vi "ci-script.vi"() -> ()   [LabVIEW 2018]
panel:
  out "error message":string
  out "Exit code":i32
  in  "arguments":string[](array[string])
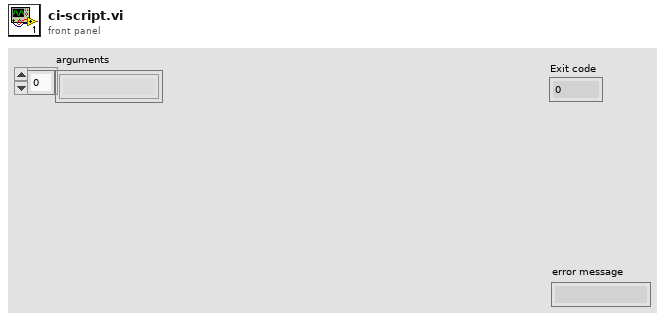
[diagram p1: front panel]
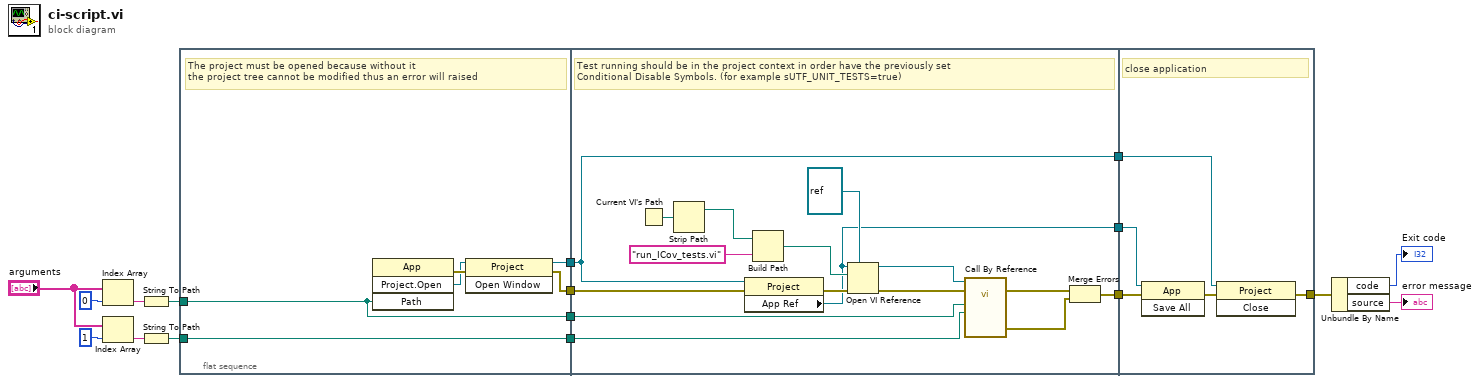
[diagram p0: block diagram]
diagram:
  n1 = Index Array(array="arguments", index=0) -> (element=w9:string)
  n2 = Index Array(array="arguments", index=1) -> (element=w7:string)
  n3 = String To Path(string=w9) -> (path=w5:path)
  n4 = String To Path(string=w7) -> (path=w4:path)
  n5 = flat-sequence {
    tunnel: w4 -> [w23]
    tunnel: w5 -> [w18]
    tunnel: [w23] -> w17
    tunnel: [w20] -> w16
    tunnel: [w19] -> w15
    tunnel: [w18] -> w14
    tunnel: w17 -> [w25]
    tunnel: w16 -> [w29]
    tunnel: w15 -> [w31]
    tunnel: [w30] -> w13
    tunnel: [w29] -> w12
    tunnel: [w28] -> w11
    tunnel: w14 -> [w26]
    tunnel: [w40] -> w3
    tunnel: w13 -> [w42]
    tunnel: w12 -> [w44]
    tunnel: w11 -> [w43]
    frame #0 {
      # "The project must be opened because without it\nthe project tree cannot be modified thus an error will raised"
      n6 = invoke class="App" method="Project.Open"("Path"=w18) -> (error out=w22:errorcluster, "Project:Open"=w21:refnum<vi>)  [unwired: 3 in, 2 out]
      n7 = invoke class="Project" method="Open Window"(reference=w21, error in=w22) -> (reference out=w20:refnum<vi>, error out=w19:errorcluster)  [unwired: 1 in, 1 out]
    }
    frame #1 {
      # "Test running should be in the project context in order have the previously set \nConditional Disable Symbols. (for example sUTF_UNIT_TESTS=true)"
      n8 = Current VI's Path() -> (path=w36:path)
      n9 = Strip Path(path=w36) -> (stripped path=w24:path)  [unwired: 1 out]
      n10 = property class="Project"(reference=w29, error in=w31) -> (error out=w37:errorcluster, "App Ref"=w28:refnum<vi>)  [unwired: 1 out]
      n11 = Build Path(base path=w24, name or relative path="run_ICov_tests.vi") -> (appended path=w34:path)
      n12 = Open VI Reference(type specifier VI Refnum (for type only)=refnum<vi> refnum, application reference (local)=w28, vi path=w34, error in (no error)=w37) -> (vi reference=w27:refnum<vi>, error out=w38:errorcluster)  [unwired: 2 in]
      n13 = call-by-ref "Call By Reference"(reference=w27, error in=w38, "<<Unit test folder>>"=w25, "<<UnitTest project path>>"=w26) -> (error out=w33:errorcluster, 0:"error out"=w32:errorcluster)  [unwired: 9 in, 1 out]
      n14 = Merge Errors(w33, w32) -> (w30:errorcluster)
    }
    frame #2 {
      # "close application"
      n15 = invoke class="App" method="Save All"(reference=w43, error in=w42) -> (error out=w41:errorcluster)  [unwired: 1 in, 2 out]
      n16 = invoke class="Project" method="Close"(reference=w44, error in=w41) -> (error out=w40:errorcluster)  [unwired: 1 in, 2 out]
    }
  }
  n17 = Unbundle By Name(w3) -> ("code"=→"Exit code":i32, "source"=→"error message":string)
